vi "Set CI Mediator Enquerer.vi"(8 "error in (no error)":errorcluster, 11 "Actor's Enqueuer":refnum<class "Message Enqueuer.lvclass">) -> (0 "error out":errorcluster)   [LabVIEW 2014]
doc: "The purpose of this VI is to share the Enqueuer with all the HTTP methods"
uses:
  <vilib>/ActorFramework/Message Enqueuer/Message Enqueuer.lvclass
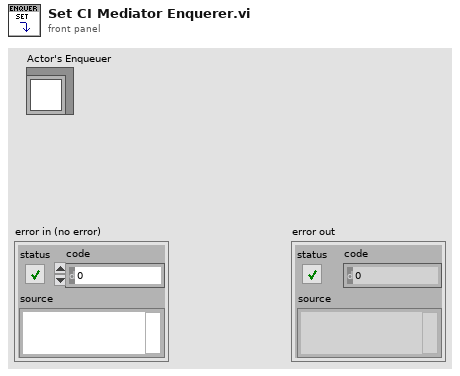
[diagram p1: front panel]
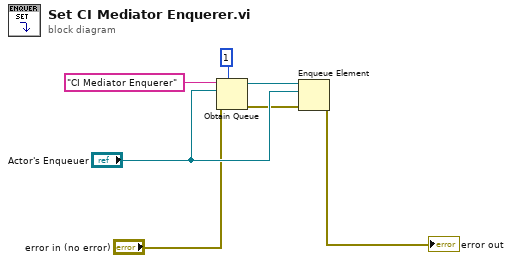
[diagram p0: block diagram]
diagram:
  n1 = Obtain Queue(max queue size (-1, unlimited)=1, name (unnamed)="CI Mediator Enquerer", element data type="Actor's Enqueuer", error in (no error)="error in (no error)") -> (queue out=w4:refnum<queue>, error out=w3:errorcluster)  [unwired: 1 in, 1 out]
  n2 = Enqueue Element(queue=w4, element="Actor's Enqueuer", error in (no error)=w3) -> (error out=→"error out":errorcluster)  [unwired: 1 in, 2 out]
